vi "CryoCooler_AVC_Open_Serial_Port.vi"(8 "error in (no error)":errorcluster, 11 "VISA Resource (write)":refnum<visa-resource-name>="COM1") -> (0 "error out":errorcluster, 3 "VISA Resource out":refnum<visa-resource-name>="COM1")   [LabVIEW 2021]
doc: "This example opens two VISA resources and configures one COM port to perform a write operation and the other COM port to perform a read operation. This VI will wait until the specified number of bytes is received at the port or until a termination character is read.\n\nThis example allows you perform diagnostic tests on your ports. You can use this example to perform a wrap-back test. Both serial ports must have the same basic configuration parameters. You can connect two of the ports using a null modem cable, which effectively connects one port's RX lines to the other port's TX lines. If you use a straight-through cable, one port's RX lines will be connected to the other port's RX lines, and you cannot communicate between the two ports."
uses:
  Serial - Settings.ctl
  <vilib>/Instr/_visa.llb/VISA Configure Serial Port (Instr).vi
panel:
  in  "End Write on Termination Character?":bool=TRUE
  # "Overview: Demonstrates the use of the VISA functions to communicate between two different serial devices.\nRequirements: NI-VISA Driver, two serial devices\nInstructions:\n1. Ensure the resources specified by VISA Resource (write) and VISA Resource (read) are valid serial devices.\n2. Connect a null modem RS-232 or RS-485/422 cable between the 2 ports.\n3. Run the VI.\n4. If your two devices are connected properly, you should see the Read String value match the Write String value."
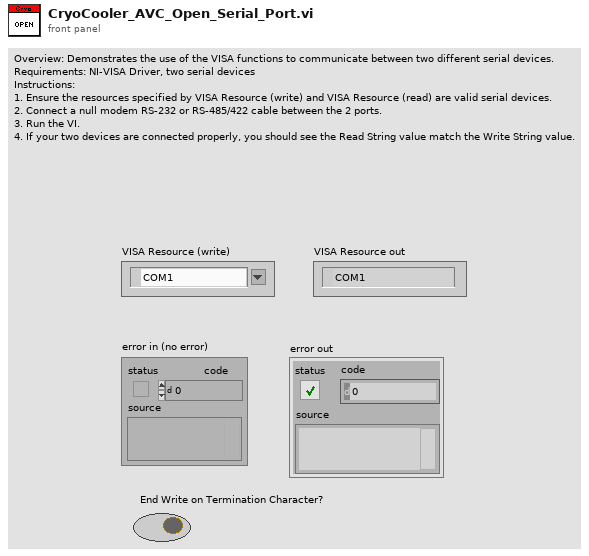
[diagram p1: front panel]
types:
  T1 = typedef "Serial - Settings.ctl" = cluster{"baud rate":u32, "data bits":u16, "parity":enum16{"None", "Odd", "Even", "Mark", "Space"}, "stop bits":u16, "flow control":u16}
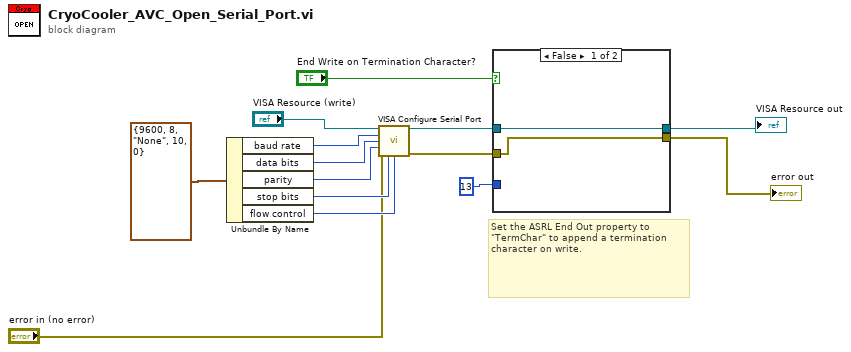
[diagram p0: block diagram]
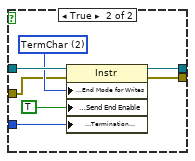
[diagram p2: hidden frame]
diagram:
  # "Set the ASRL End Out property to \"TermChar\" to append a termination character on write."
  n1 = Unbundle By Name(T1 {"baud rate"=9600, "data bits"=8, "parity"=enum."None", "stop bits"=10, "flow control"=0} ("Serial Settings (write)")) -> ("baud rate"=w9:u32, "data bits"=w8:u16, "parity"=w7:enum16{"None", "Odd", "Even", "Mark", "Space"}, "stop bits"=w6:u16, "flow control"=w5:u16)
  n2 = call-poly "VISA Configure Serial Port"("VISA resource name"="VISA Resource (write)", "baud rate (9600)"=w9, "data bits (8)"=w8, "parity (0:none)"=w7, "error in (no error)"="error in (no error)", "stop bits (10: 1 bit)"=w6, "flow control (0:none)"=w5) -> ("VISA resource name out"=w13:refnum<visa-resource-name>, "error out"=w2:errorcluster)  [unwired: 2 in, 5 out]
  n3 = case shown="False" "End Write on Termination Character?" {
    tunnel: w13 -> [w16 w23]
    tunnel: [w16 w22] -> w3
    tunnel: [w15 w21] -> w1
    tunnel: u8 13 ("Termination Character") -> [_ w19]
    tunnel: w2 -> [w15 w17]
    frame False {
    }
    frame True {
      w20 = u16 2 items=["None", "LastBit", "TermChar", "Break"] ("Serial Settings:Serial End Mode for Writes")
      n4 = property class="Instr"(reference=w23, error in=w17, "Serial Settings:End Mode for Writes"=w20, "Message Based Settings:Send End Enable"=TRUE, "Message Based Settings:Termination Character"=w19) -> (reference out=w22:refnum<visa-resource-name>, error out=w21:errorcluster)
    }
  }
  "VISA Resource out" <- w3
  "error out" <- w1
